vi "Read Rectangle.vi"(8 "error in (no error)":errorcluster, 11 "Canvas in":refnum<class "Drawer .Net.lvclass">) -> (0 "error out":errorcluster, 2 "Rectangle":refnum<k24>, 3 "Canvas out":refnum<class "Drawer .Net.lvclass">)   [LabVIEW 2023, in "Glyph .NET Drawer.lvlib" / "Drawer .Net.lvclass"]
uses:
  Drawer .Net.lvclass
  System.Drawing
  Drawer .Net.lvclass/Drawer .Net.ctl
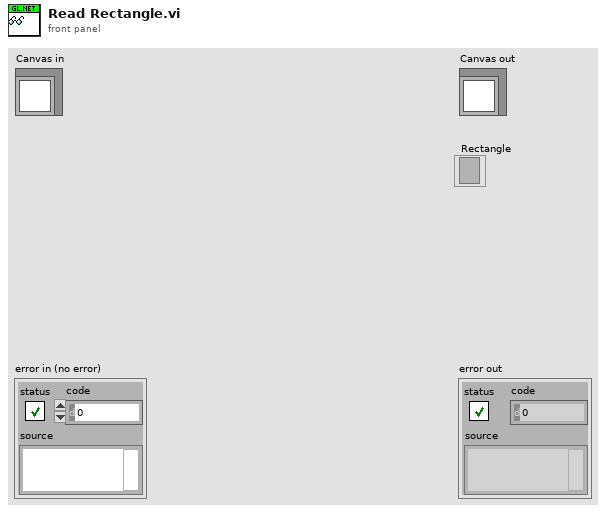
[diagram p1: front panel]
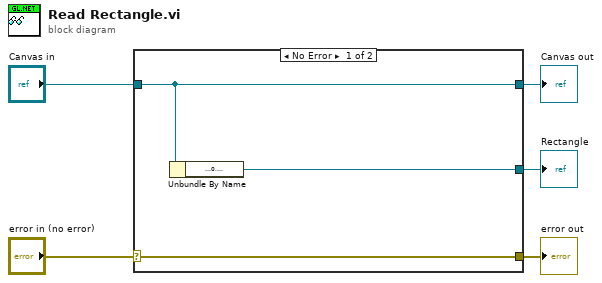
[diagram p0: block diagram]
diagram:
  n1 = case shown="No Error" "error in (no error)" {
    selector: "error in (no error)" -> [w8 w9]
    tunnel: [w8 w9] -> w4
    tunnel: [w7 w10] -> w2
    tunnel: "Canvas in" -> [w7 w10]
    tunnel: [w6 _] -> w1
    frame No Error {
      n2 = Unbundle By Name(w7) -> ("Rectangle"=w6:refnum<k24>)
    }
    frame Error {
    }
  }
  "error out" <- w4
  "Canvas out" <- w2
  "Rectangle" <- w1
